vi "OpenXL_Workbook.vi"(8 "error in":errorcluster, 10 "path":path, 11 "Refnum Cluster In":T1) -> (0 "error out":errorcluster, 3 "Refnum Cluster Out":T2)   [LabVIEW 2015]
doc: "This VI opens an Excel Workbook. Pair this VI with CloseXL_Workbook.vi."
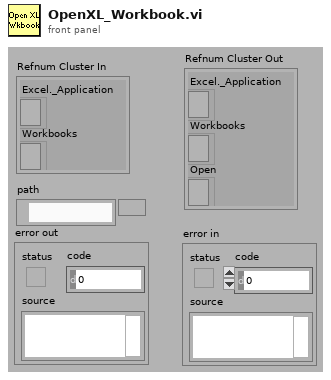
[diagram p1: front panel]
types:
  T1 = cluster{"Excel._Application":refnum<k7>, "Workbooks":refnum<k7>}
  T2 = cluster{"Excel._Application":refnum<k7>, "Workbooks":refnum<k7>, "Open":refnum<k7>}
  T3 = enum32{"existing file", "new file", "new or existing file", "existing dir", "new dir", "new or existing dir", "existing file (use LLBs)", "new file (use LLBs)", "new or existing file (use LLBs)", "new or existing file or directory (use LLBs)"}
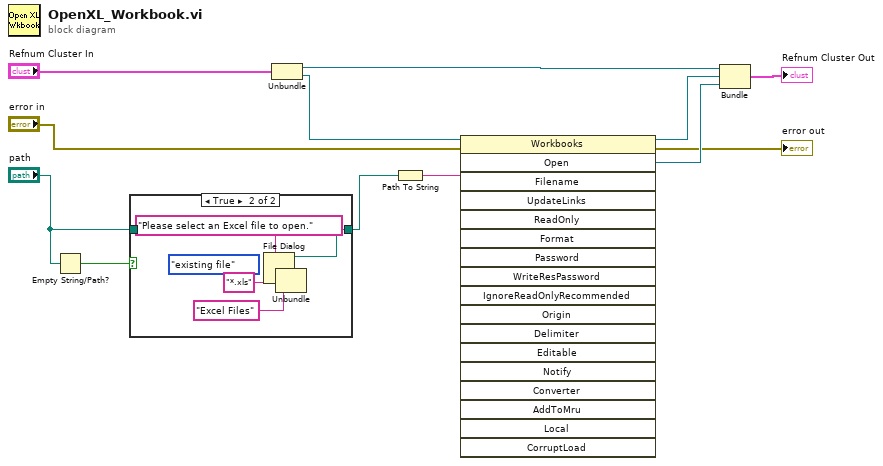
[diagram p0: block diagram]
diagram:
  n1 = Empty String/Path?(string/path="path") -> (empty?=w3:bool)
  n2 = case shown="True" w3 {
    tunnel: "path" -> [w13 _]
    tunnel: [w13 w18] -> w1
    frame False {
    }
    frame True {
      (unwired) T3."existing file" ("select mode (2)")
      n3 = File Dialog(4:"Excel Files" ("pattern label"), 6:"*.xls" ("pattern"), 7:"Please select an Excel file to open." ("prompt")) -> (0:w14:errorcluster, 3:w18:path)  [unwired: 4 in, 2 out]
      n4 = Unbundle(w14) -> ()  [unwired: 3 out]
    }
  }
  n5 = Unbundle("Refnum Cluster In") -> ("Excel._Application"=w9:refnum<k7>, "Workbooks"=w5:refnum<k7>)
  n6 = Path To String(path=w1) -> (string=w7:string)
  n7 = invoke class="Workbooks" method="Open"(reference=w5, error in="error in", "Filename"=w7) -> (reference out=w10:refnum<k7>, error out=→"error out":errorcluster, "Open"=w11:refnum<k7>)  [unwired: 15 in, 15 out]
  n8 = Bundle("Excel._Application"=w9, "Workbooks"=w10, "Open"=w11) -> (→"Refnum Cluster Out":T2)  [unwired: 1 in]
